vi "Remove the Repeat Element.vi"() -> ()   [LabVIEW 2015]
panel:
  in  "Name List":string[](array[string])
  in  "Str1 2":string
  out "Str 3":cluster{"Str1":string, "St2":string}
  out "duplicate variant":variant
  in  "Array":cluster{"Str1":string, "St2":string}[](array[cluster])=[{"Str1"="A123", "St2"="B123"}, {"Str1"="A456", "St2"="B456"}, {"Str1"="A789", "St2"="B789"}]
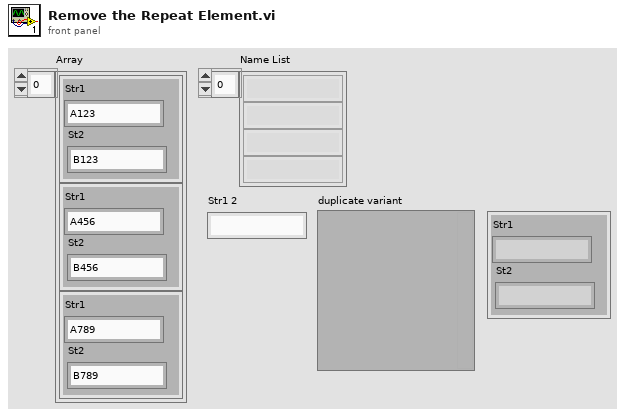
[diagram p1: front panel]
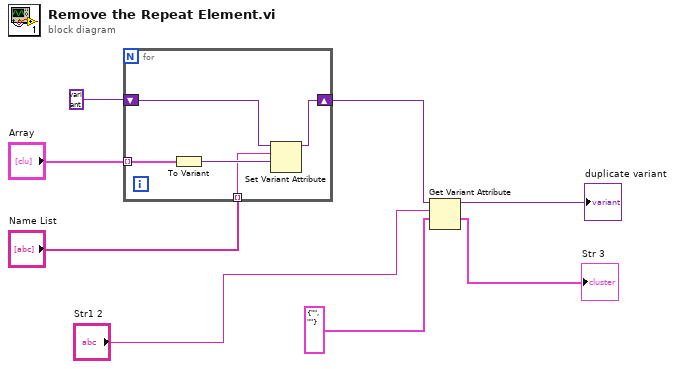
[diagram p0: block diagram]
diagram:
  n1 = for {
    tunnel: "Name List" -> [w12] mode=indexing
    tunnel: "Array" -> [w11] mode=indexing
    shift-right: [w9] -> w4
    shift-left: variant -> [w10]
    n2 = To Variant(anything=w11) -> (Variant=w13:variant)
    n3 = Set Variant Attribute(Variant=w10, name=w12, value=w13) -> (Variant out=w9:variant)  [unwired: 1 in, 2 out]
  }
  n4 = Get Variant Attribute(Variant=w4, name="Str1 2", default value (empty Variant)=cluster{"Str1":string, "St2":string} {"Str1"="", "St2"=""} ("Str 2")) -> (duplicate Variant=→"duplicate variant":variant, value=→"Str 3":cluster{"Str1":string, "St2":string})  [unwired: 1 in, 2 out]
